vi "Import in Place.vi"(8 "error in":errorcluster, 10 "path":path, 11 "item ref":T1 format="%.0x") -> (0 "error out":errorcluster, 3 "new item ref":T1 format="%.0x")   [LabVIEW 2027, in "Custom Device Serialization.lvlib"]
uses:
  Custom Device Serialization.lvlib
  <vilib>/NI VeriStand/Custom Device API/Custom Device Item Ref.ctl
  <vilib>/NI VeriStand/Custom Device API/Custom Device API.lvlib
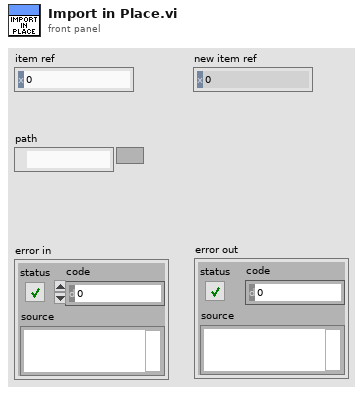
[diagram p1: front panel]
types:
  T1 = typedef "Custom Device API.lvlib/Custom Device Item Ref.ctl" = u64
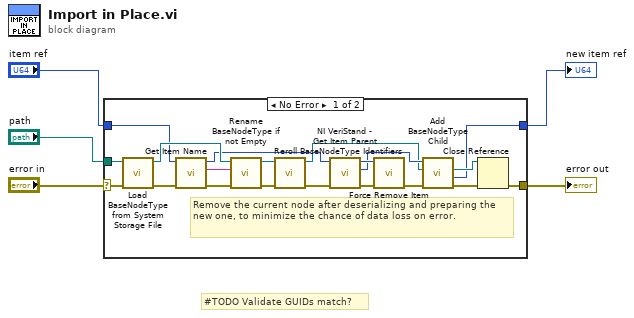
[diagram p0: block diagram]
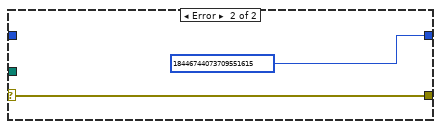
[diagram p2: hidden frame]
diagram:
  # "#TODO Validate GUIDs match?"
  n1 = case shown="No Error" "error in" {
    selector: "error in" -> [w24 w27]
    tunnel: "path" -> [w25 _]
    tunnel: [w21 w27] -> w3
    tunnel: "item ref" -> [w7 _]
    tunnel: [w20 T1 18446744073709551615 ("child ref")] -> w2
    frame No Error {
      # "Remove the current node after deserializing and preparing the new one, to minimize the chance of data loss on error."
      n2 = call "Load BaseNodeType from System Storage File.vi"("error in (no error)"=w24, "path"=w25) -> ("error out"=w11:errorcluster, "NationalInstruments.VeriStand.SystemStorage.BaseNodeType"=w10:refnum<k39>)  [unwired: 8 in]
      n3 = call "Get Item Name.vi"("error in"=w11, "item ref in"=w7) -> ("error out"=w9:errorcluster, "name"=w8:string, "item ref out"=w6:T1)  [unwired: 7 in]
      n4 = call "Rename BaseNodeType if not Empty.vi"("error in"=w9, "name"=w8, "NationalInstruments.VeriStand.SystemStorage.BaseNodeType"=w10) -> ("error out"=w19:errorcluster, "NationalInstruments.VeriStand.SystemStorage.BaseNodeType"=w18:refnum<k39>)  [unwired: 7 in]
      n5 = call "Reroll BaseNodeType Identifiers.vi"("error in"=w19, "NationalInstruments.VeriStand.SystemStorage.BaseNodeType"=w18) -> ("error out"=w17:errorcluster, "NationalInstruments.VeriStand.SystemStorage.BaseNodeType"=w12:refnum<k39>)  [unwired: 8 in]
      n6 = call <vilib>:"NI VeriStand - Get Item Parent.vi"("error in (no error)"=w17, "Item Ref in"=w6) -> ("error out"=w15:errorcluster, "Parent Ref"=w13:T1, "Item Ref out"=w14:T1)  [unwired: 6 in, 1 out]
      n7 = call "Force Remove Item.vi"("error in"=w15, "item ref"=w14) -> ("error out"=w16:errorcluster)  [unwired: 9 in]
      n8 = call "Add BaseNodeType Child.vi"("error in"=w16, "NationalInstruments.VeriStand.SystemStorage.BaseNodeType"=w12, "parent ref in"=w13) -> ("error out"=w22:errorcluster, "child ref"=w20:T1, "NationalInstruments.VeriStand.SystemStorage.BaseNodeType"=w23:refnum<k39>)  [unwired: 5 in, 1 out]
      n9 = Close Reference(reference=w23, error in (no error)=w22) -> (error out=w21:errorcluster)
    }
    frame Error {
    }
  }
  "error out" <- w3
  "new item ref" <- w2
